vi "Close handle.vi"(1 "Device Handle":u32) -> (0 "Error":errorcluster)   [LabVIEW 2014]
uses:
  Program Files (x86)/Coherent/HOPS/CohrHOPS.dll
panel:
  # "PN 04/11/2014"
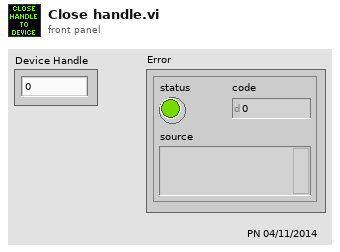
[diagram p1: front panel]
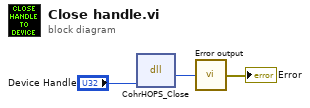
[diagram p0: block diagram]
diagram:
  n1 = dll-call lib="C:/Program Files (x86)/Coherent/HOPS/CohrHOPS.dll" fn="CohrHOPS_Close"("handle"="Device Handle") -> ("return type"=w2:i32)  [unwired: 4 in, 2 out]
  n2 = call "Error output.vi"("I32 err code"=w2) -> ("Error Out"=→"Error":errorcluster)
